vi "OSF Append Wiki.vi"(6 "content":string, 7 "OSF API URL":string="https://api.osf.io/v2/", 8 "error in":errorcluster, 10 "Wiki  ID":string, 11 "client handle":T2) -> (0 "error out":errorcluster, 2 "Responce body":string, 3 "client handle out":T2)   [LabVIEW 2020]
uses:
  <vilib>/httpClient/ClientHandle.ctl
  55103850-15ef-4a18-9388-7b0eadcdd449.vi
  <vilib>/JDP Science/JSONtext/Variant to JSON Text.vi
  <vilib>/httpClient/POSTBuffer.vi
  <vilib>/JDP Science/JSONtext/LVClass Serializer/JSONtext LVClass Serializer.lvclass
  <vilib>/httpClient/LabVIEWHTTPClient.lvlib
  <vilib>/JDP Science/JSONtext/JSONtext.lvlib
panel:
  out "Display Text":string
  out "Content":string
  out "Get responce":string
  in  "OSF Wiki Content":T1={"data"={"id"="", "type"="wiki-versions", "attributes"={"content"=""}}}
  out "Puject  JSON":string
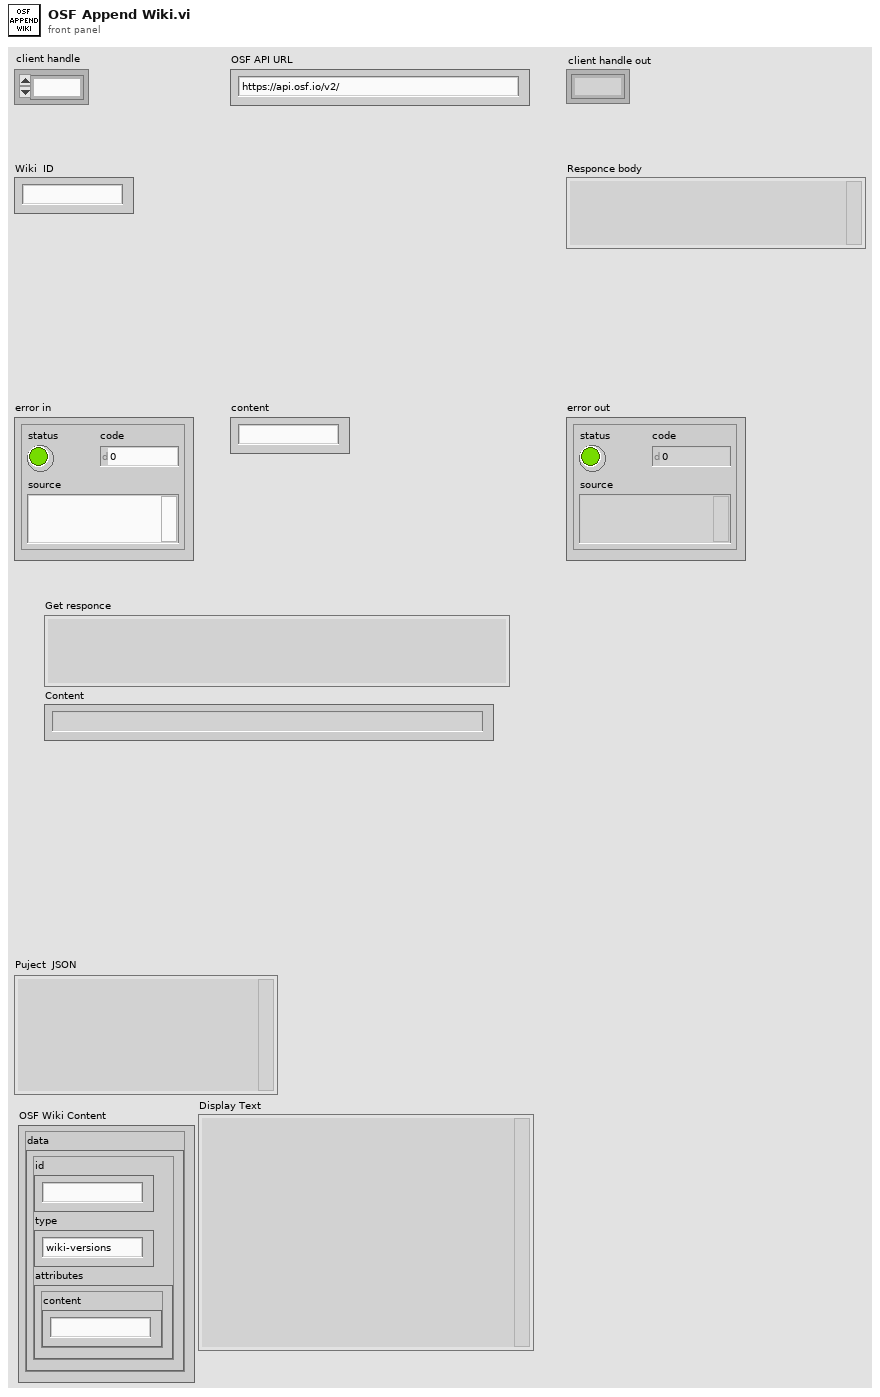
[diagram p1: front panel]
types:
  T1 = cluster{"data":cluster{"id":string, "type":string, "attributes":cluster{"content":string}}}
  T2 = typedef "LabVIEWHTTPClient.lvlib/ClientHandle.ctl" = refnum<k1>
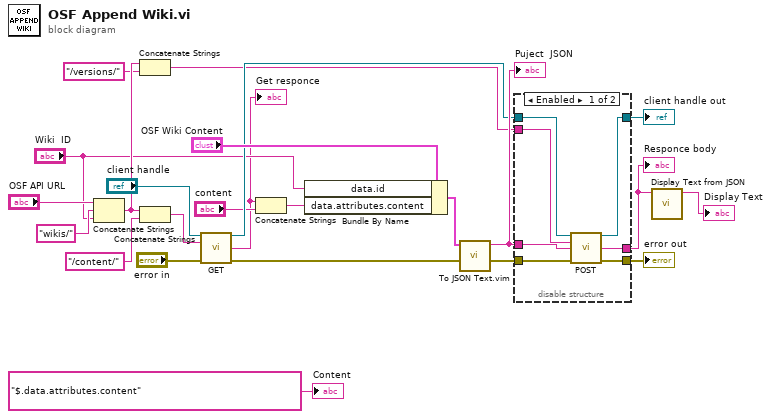
[diagram p0: block diagram]
diagram:
  n1 = Concatenate Strings("OSF API URL", "wikis/", "Wiki  ID") -> (w8:string)
  n2 = Concatenate Strings(w8, "/versions/" ("string")) -> (w7:string)
  n3 = Concatenate Strings(w8, "/content/" ("string")) -> (w9:string)
  n4 = call <vilib>:"GET.vi"("client handle"="client handle", "url"=w9, "error in (no error)"="error in") -> ("client handle out"=w14:T2, "body"=w2:string, "error out"=w13:errorcluster)  [unwired: 9 in, 1 out]
  "Get responce" <- w2
  n5 = Concatenate Strings(w2, "content") -> (w3:string)
  n6 = Bundle By Name(cluster="OSF Wiki Content", "data.id"="Wiki  ID", "data.attributes.content"=w3) -> (w24:T1)
  n7 = call "To JSON Text.vim"("error in (no error)"=w13, "Anything"=w24) -> ("error out"=w20:errorcluster, "<JSON>"=w17:string)  [unwired: 8 in]
  "Puject  JSON" <- w17
  n8 = disable-structure shown="Enabled" {
    disable-tunnel: [w31 w32] -> w23
    disable-tunnel: w7 -> [w30 _]
    disable-tunnel: w20 -> [w29 w33]
    disable-tunnel: [w28 w33] -> w19
    disable-tunnel: [w27 _] -> w1
    disable-tunnel: w17 -> [w26 _]
    disable-tunnel: w14 -> [w25 w32]
    frame Enabled {
      n9 = call-poly <vilib>:"POST.vi"("client handle"=w25, "url"=w30, "buffer"=w26, "error in (no error)"=w29) -> ("client handle out"=w31:T2, "body"=w27:string, "error out"=w28:errorcluster)  [unwired: 8 in, 1 out]
    }
    frame Disabled {
    }
  }
  "error out" <- w19
  "client handle out" <- w23
  "Responce body" <- w1
  n10 = call <vilib>:"Display Text from JSON.vi"("Input JSON"=w1) -> ("Display Text"=→"Display Text":string)  [unwired: 8 in, 2 out]
  "Content" <- "$.data.attributes.content"
